vi "Shutdown.vi"(8 "error in (no error)":errorcluster, 11 "Simulated Actuator in":refnum<class "Simulated Actuator.lvclass">) -> (0 "error out":errorcluster, 3 "Simulated Actuator out":refnum<class "Simulated Actuator.lvclass">)   [LabVIEW 2020, in "Simulated Actuator.lvclass"]
uses:
  Simulated Actuator.lvclass
  Simulated Actuator.lvclass/Simulated Actuator.ctl
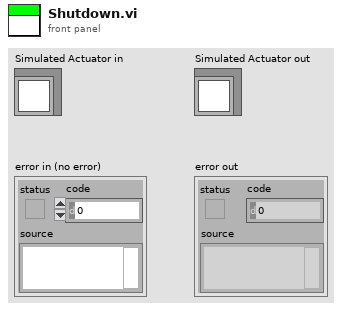
[diagram p1: front panel]
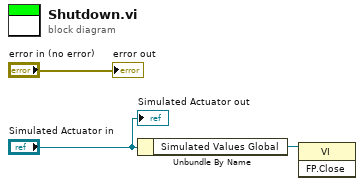
[diagram p0: block diagram]
diagram:
  n1 = Unbundle By Name("Simulated Actuator in") -> ("Simulated Values Global"=w2:refnum<vi>)
  n2 = invoke class="VI" method="FP.Close"(reference=w2) -> ()  [unwired: 2 in, 3 out]
  "error out" <- "error in (no error)"
  "Simulated Actuator out" <- "Simulated Actuator in"
